vi "主界面.vi"() -> ()   [LabVIEW 2016, in "main.lvlib"]
uses:
  main.lvlib
  <vilib>/Utility/miscctls.llb/LVPointTypeDef.ctl
  <vilib>/Plasmionique/MB Master/MB_Master/MB_Master.lvclass
  DST800/DST800.lvlib
  elevator/elevator.lvlib
  EXO2/EXO2.lvlib
  DAM395CF/DAM395CF.lvlib
  <vilib>/ptbypt/NI_PtbyPt.lvlib
  bbe/bbe.lvlib
  NAQ_DO/NAQ_DO.lvlib
panel:
  out "循环次数":u32
  in  "急停按钮":bool
  out "告警信息":string
  out "运行状态":bool
  out "位置变化值":dbl
  out "编码器计数值":u16
  in  "停止按钮":bool
  in  "启动":bool
  in  "剖面视图":bool
  out "日志":string
  in  "监测数据":i32(listbox)
  out "声纳通讯":bool
  out "仪器通讯":bool
  out "IO通讯":bool
  out "多参数电源":bool caption="仪器电源"
  out "剖面下降":bool
  out "剖面上升":bool
  in  "调试":bool
  in  "设置":bool
  out "仪器位置":dbl format="%#_6f m"
  out "湖面水深":dbl format="%#_6f m"
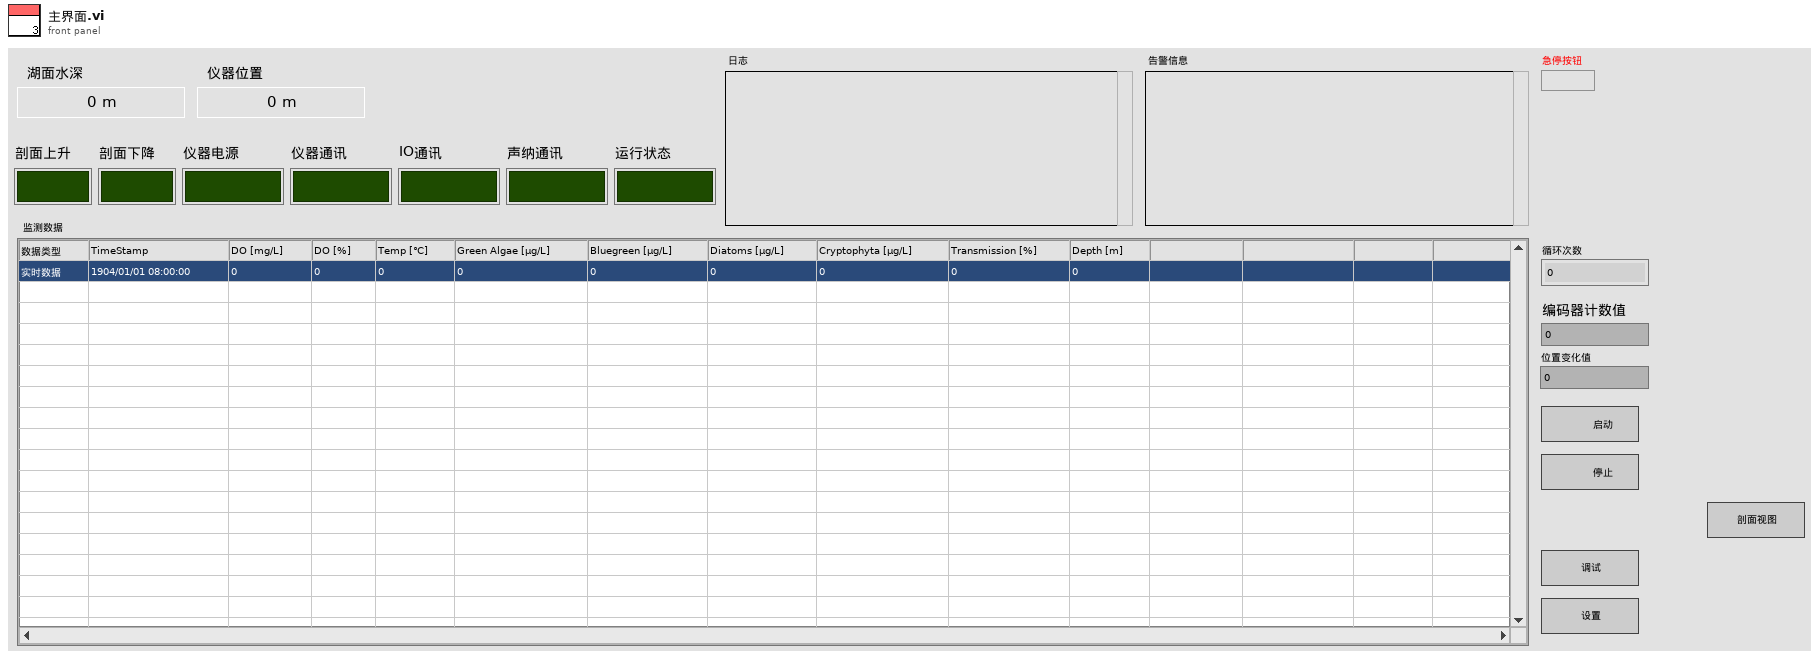
[diagram p1: front panel]
types:
  T1 = enum16{"open", "poll", "close", "run", "stop", "shutdown"}
  T2 = typedef "LVPointTypeDef.ctl" = cluster{"Horizontal":i16, "Vertical":i16}
  T3 = cluster{"Time":timestamp, "Temp":dbl, "SpCond":dbl, "Cond":dbl, "Sal":dbl, "TDS":dbl, "pH":dbl, "pH mV":dbl, "orp":dbl, "ODO %":dbl, "ODO mg/L":dbl, "Turb":dbl, "Chl":dbl, "Depth":dbl}
  T4 = cluster{"时间":timestamp, "Temp [℃]":dbl, "Green Algae [μg/L]":dbl, "Bluegreen [μg/L]":dbl, "Diatoms [μg/L]":dbl, "Cryptophyta [μg/L]":dbl, "Transmission [%]":dbl, "Depth [m]":dbl}
  T5 = cluster{"编码器工程变换系数_计数值":dbl, "编码器工程变换系数_工程值":dbl}
  T6 = typedef "checkbox.ctl" = bool
  T7 = typedef "剖面数据_EXO2.ctl" = cluster{"时间":timestamp, "测量模式":string, "数据类型":string, "数据标识":string, "湖面水深":sgl, "缆绳下放长度":sgl, "层数":u16, "row":u16, "水温":sgl, "比电导率":sgl, "电导率":sgl, "盐度":sgl, "总溶解固体":sgl, "pH":sgl, "pHmV":sgl, "ORP":sgl, "饱和度":sgl, "DO":sgl, "浊度":sgl, "叶绿素a":sgl, "水深":sgl}
  T8 = typedef "剖面数据_bbe_NAQDO.ctl" = cluster{"时间":timestamp, "测量模式":string, "数据类型":string, "数据标识":string, "湖面水深":sgl, "缆绳下放长度":sgl, "层数":u16, "row":u16, "水温":sgl, "DO":sgl, "饱和度":sgl, "绿藻":sgl, "蓝藻":sgl, "硅甲藻":sgl, "隐藻":sgl, "透光率":sgl, "水深":sgl}
  T9 = cluster{"水温":sgl, "比电导率":sgl, "电导率":sgl, "盐度":sgl, "总溶解固体":sgl, "pH":sgl, "pHmV":sgl, "ORP":sgl, "饱和度":sgl, "DO":sgl, "浊度":sgl, "叶绿素a":sgl, "水深":sgl}
  T10 = cluster{"时间标识":timestamp, "DO [mg/L]":dbl, "DO [%]":dbl}
  T11 = cluster{"水温":sgl, "DO":sgl, "饱和度":sgl, "绿藻":sgl, "蓝藻":sgl, "硅甲藻":sgl, "隐藻":sgl, "透光率":sgl, "水深":sgl}
  T12 = typedef "LVDateTimeRec.ctl" = cluster{"秒数的小数部分":dbl, "秒":i32, "分":i32, "时":i32, "日":i32, "月":i32, "年":i32, "天数（周）":i32, "天数（年）":i32, "DST":i32}
  T13 = cluster{"baud rate (bps)":u32, "stop bits":u16, "parity":u16, "flow control":u16, "timeout":u32, "retries":i32}
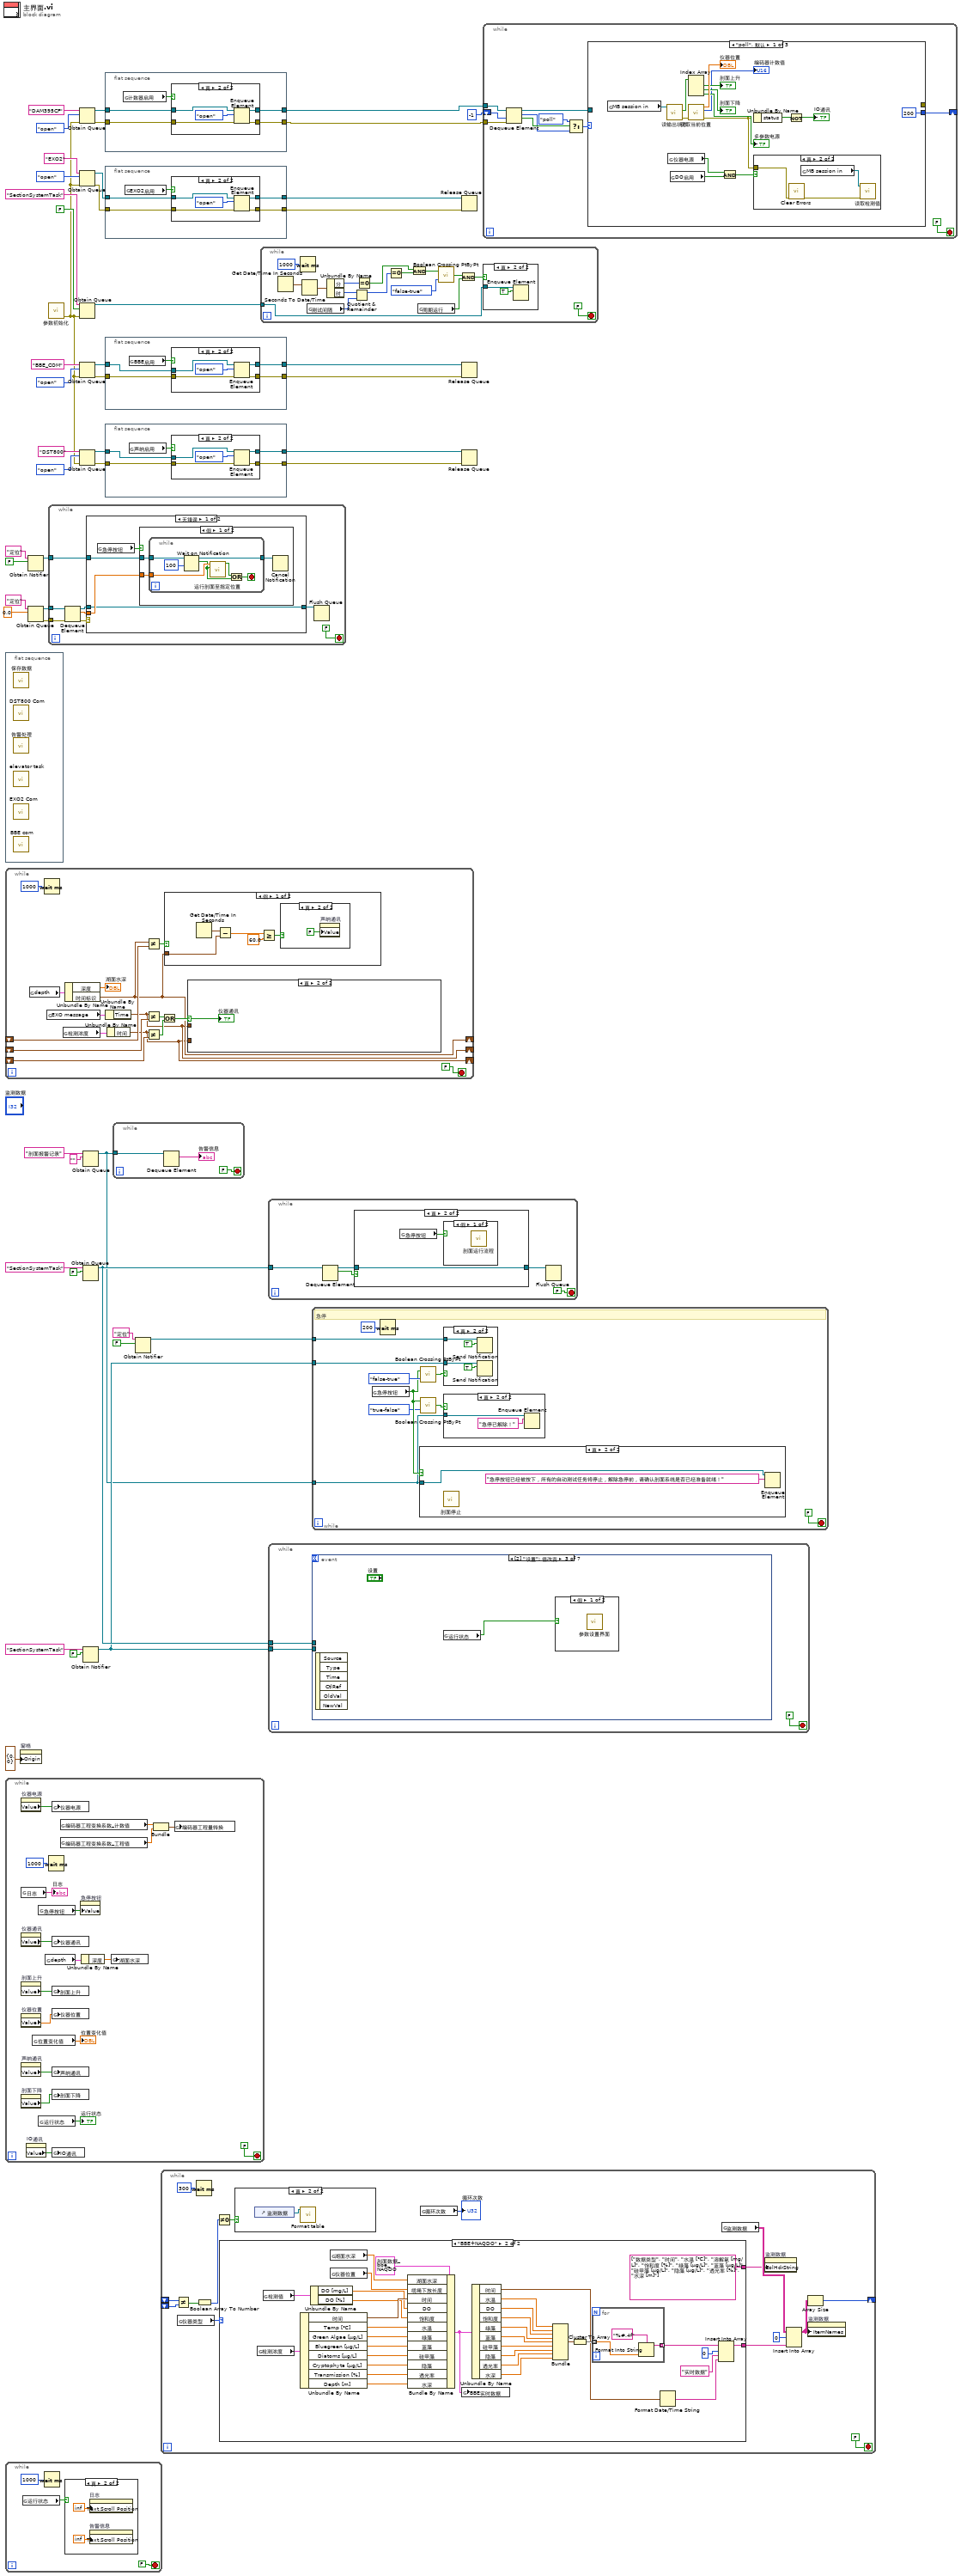
[diagram p0: block diagram]
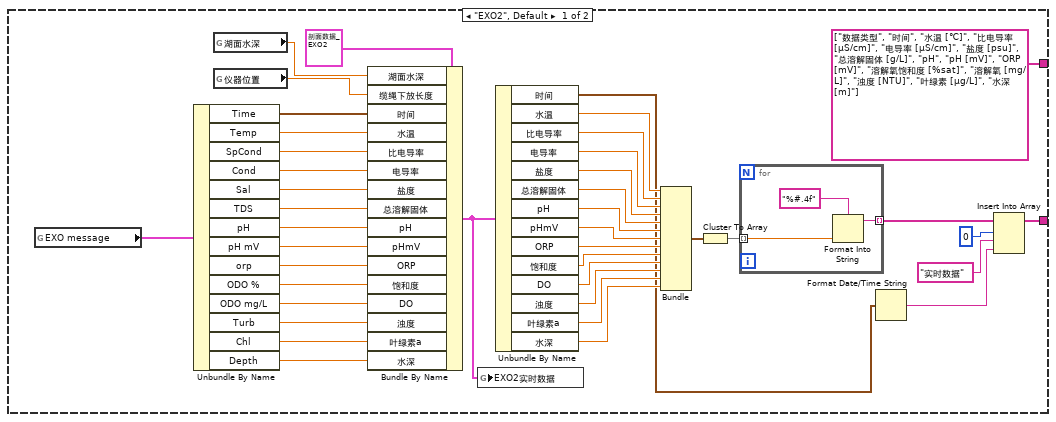
[diagram p6: hidden frame]
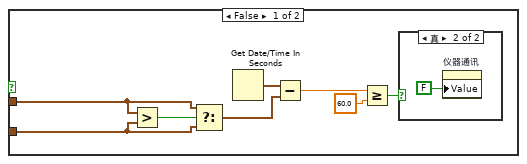
[diagram p14: hidden frame]
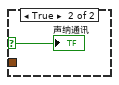
[diagram p17: hidden frame]
diagram:
  n1 = flat-sequence {
    frame #0 {
      n2 = call "保存数据.vi"() -> ()  [unwired: 12 in]
      n3 = call "DST800 Com.vi"() -> ()  [unwired: 12 in]
      n4 = call "告警处理.vi"() -> ()  [unwired: 12 in]
      n5 = call "elevator task.vi"() -> ()  [unwired: 12 in]
      n6 = call "EXO2 Com.vi"() -> ()  [unwired: 12 in]
      n7 = call "BBE com.vi"() -> ()  [unwired: 12 in]
    }
  }
  n8 = while {
    shift-right: [w52] -> _
    shift-left: _ -> [w62]
    shift-right: [w51] -> _
    shift-left: _ -> [w59]
    shift-right: [w50] -> _
    shift-left: _ -> [w56]
    stop <- FALSE stop-if-true
    n9 = global read "DST800全局变量.vi" "depth"() -> (w64:cluster{"时间标识":timestamp, "深度":dbl})
    n10 = Wait (ms)(milliseconds to wait=u32 1000 ("等待时间（毫秒）")) -> ()  [unwired: 1 out]
    n11 = global read "EXO2全局变量.vi" "EXO message"() -> (w60:T3)
    n12 = global read "过程变量.vi" "检测浓度"() -> (w57:T4)
    n13 = Unbundle By Name(w64) -> ("深度"=→"湖面水深":dbl, "时间标识"=w52:timestamp)
    n14 = Unbundle By Name(w60) -> ("Time"=w51:timestamp)
    n15 = Unbundle By Name(w57) -> ("时间"=w50:timestamp)
    n16 = Not Equal?(x=w52, y=w62) -> (x != y?=w54:bool)
    n17 = Not Equal?(x=w51, y=w59) -> (x != y?=w58:bool)
    n18 = Not Equal?(x=w50, y=w56) -> (x != y?=w55:bool)
    n19 = Or(x=w58, y=w55) -> (x .or. y?=w53:bool)
    n20 = case shown="假" w54 {
      selector: w54 -> [_ w82]
      tunnel: w52 -> [w80 _]
      frame False {
        n21 = Get Date/Time In Seconds() -> (seconds since 1Jan1904=w79:timestamp)
        n22 = Subtract(x=w79, y=w80) -> (x-y=w78:dbl)
        n23 = Greater Or Equal?(x=w78, y=60.0) -> (x >= y?=w76:bool)
        n24 = case shown="真" w76 {
          frame False {
          }
          frame True {
            n25 = property on="声纳通讯" class="Bool (严格)"("Value"=FALSE ("声纳通讯")) -> ()  [unwired: 2 in, 2 out]
          }
        }
      }
      frame True {
        "声纳通讯" <- w82
      }
    }
    n26 = case shown="真" w53 {
      selector: w53 -> [_ w75]
      tunnel: w51 -> [w68 _]
      tunnel: w50 -> [w67 _]
      frame False {
        n27 = Greater?(x=w68, y=w67) -> (0:w69:bool)
        n28 = Select(t=w68, s=w69, f=w67) -> (s? t:f=w66:timestamp)
        n29 = Get Date/Time In Seconds() -> (seconds since 1Jan1904=w70:timestamp)
        n30 = Subtract(x=w70, y=w66) -> (x-y=w71:dbl)
        n31 = Greater Or Equal?(x=w71, y=60.0) -> (x >= y?=w73:bool)
        n32 = case shown="真" w73 {
          frame False {
          }
          frame True {
            n33 = property on="仪器通讯" class="Bool (严格)"("Value"=FALSE ("声纳通讯")) -> ()  [unwired: 2 in, 2 out]
          }
        }
      }
      frame True {
        "仪器通讯" <- w75
      }
    }
  }
  n34 = while {
    stop <- FALSE stop-if-true
    n35 = property on="仪器电源" class="Bool (严格)"() -> ("Value"=w84:bool)  [unwired: 2 in, 2 out]
    n36 = global read "全局非断电保持变量.vi" "日志"() -> (→"日志":string)
    n37 = property on="仪器通讯" class="Bool (严格)"() -> ("Value"=w93:bool)  [unwired: 2 in, 2 out]
    n38 = property on="剖面上升" class="Bool (严格)"() -> ("Value"=w95:bool)  [unwired: 2 in, 2 out]
    n39 = property on="仪器位置" class="DigNum (严格)"() -> ("Value"=w92:dbl)  [unwired: 2 in, 2 out]
    n40 = property on="声纳通讯" class="Bool (严格)"() -> ("Value"=w94:bool)  [unwired: 2 in, 2 out]
    n41 = property on="剖面下降" class="Bool (严格)"() -> ("Value"=w96:bool)  [unwired: 2 in, 2 out]
    n42 = property on="IO通讯" class="Bool (严格)"() -> ("Value"=w97:bool)  [unwired: 2 in, 2 out]
    n43 = global read "全局非断电保持变量.vi" "位置变化值"() -> (→"位置变化值":dbl)
    n44 = global read "全局非断电保持变量.vi" "急停按钮"() -> (w83:bool)
    n45 = global read "全局非断电保持变量.vi" "运行状态"() -> (→"运行状态":bool)
    n46 = global read "DST800全局变量.vi" "depth"() -> (w99:cluster{"时间标识":timestamp, "深度":dbl})
    n47 = Wait (ms)(milliseconds to wait=u32 1000 ("等待时间（毫秒）")) -> ()  [unwired: 1 out]
    n48 = global write "全局非断电保持变量.vi" "仪器电源"(w84) -> ()
    n49 = global write "全局非断电保持变量.vi" "仪器通讯"(w93) -> ()
    n50 = global write "全局非断电保持变量.vi" "剖面上升"(w95) -> ()
    n51 = global write "全局非断电保持变量.vi" "仪器位置"(w92) -> ()
    n52 = global write "全局非断电保持变量.vi" "声纳通讯"(w94) -> ()
    n53 = global write "全局非断电保持变量.vi" "剖面下降"(w96) -> ()
    n54 = global write "全局非断电保持变量.vi" "IO通讯"(w97) -> ()
    n55 = global read "全局断电保存变量.vi" "编码器工程变换系数_计数值"() -> (w89:dbl)
    n56 = global read "全局断电保存变量.vi" "编码器工程变换系数_工程值"() -> (w88:dbl)
    n57 = property on="急停按钮" class="Bool (严格)"("Value"=w83) -> ()  [unwired: 2 in, 2 out]
    n58 = Unbundle By Name(w99) -> ("深度"=w98:dbl)
    n59 = global write "全局非断电保持变量.vi" "湖面水深"(w98) -> ()
    n60 = Bundle("编码器工程变换系数_计数值"=w89, "编码器工程变换系数_工程值"=w88) -> (w87:T5)  [unwired: 1 in]
    n61 = global write "elevator 全局变量.vi" "编码器工程量转换"(w87) -> ()
  }
  n62 = while {
    stop <- FALSE stop-if-true
    n63 = global read "全局非断电保持变量.vi" "运行状态"() -> (w101:bool)
    n64 = Wait (ms)(milliseconds to wait=u32 1000 ("等待时间（毫秒）")) -> ()  [unwired: 1 out]
    n65 = case shown="真" w101 {
      frame False {
      }
      frame True {
        n66 = property on="日志" class="Str"("Text.Scroll Position"=inf) -> ()  [unwired: 2 in, 2 out]
        n67 = property on="告警信息" class="Str"("Text.Scroll Position"=inf) -> ()  [unwired: 2 in, 2 out]
      }
    }
  }
  n68 = property on="窗格" class="Pane"("Origin"=T2 {"Horizontal"=0, "Vertical"=0} ("原点")) -> ()  [unwired: 2 in, 2 out]
  n69 = Obtain Notifier(name (unnamed)="定位" ("名称（未命名）"), notification data type=FALSE) -> (notifier out=w18:refnum<notifier>)  [unwired: 2 in, 2 out]
  n70 = Obtain Queue(name (unnamed)="定位" ("名称（未命名）"), element data type=0.0) -> (queue out=w22:refnum<queue>, error out=w21:errorcluster)  [unwired: 3 in, 1 out]
  n71 = call "参数初始化.vi"() -> ("error out"=w6:errorcluster)  [unwired: 11 in]
  n72 = while {
    tunnel: w22 -> [w113]
    tunnel: w21 -> [w112]
    tunnel: w18 -> [w109]
    stop <- FALSE stop-if-true
    n73 = Dequeue Element(queue=w113, error in (no error)=w112) -> (queue out=w108:refnum<queue>, element=w110:dbl, error out=w111:errorcluster)  [unwired: 1 in, 1 out]
    n74 = case shown="无错误" w111 {
      tunnel: w110 -> [w117 _]
      tunnel: w109 -> [w116 _]
      tunnel: [w115 w128] -> w107
      tunnel: w108 -> [w115 w128]
      frame No Error {
        n75 = global read "全局非断电保持变量.vi" "急停按钮"() -> (w114:bool)
        n76 = case shown="假" w114 {
          tunnel: w117 -> [w120 _]
          tunnel: w116 -> [w119 _]
          frame False {
            n77 = while {
              tunnel: w120 -> [w127]
              tunnel: w119 -> [w126]
              tunnel: [w122] -> w118
              stop <- w124 stop-if-true
              n78 = Wait on Notification(notifier=w126, timeout in ms (-1)=100 ("超时毫秒(-1)")) -> (notifier out=w122:refnum<notifier>, notification=w121:bool)  [unwired: 2 in, 2 out]
              n79 = call "运行剖面至指定位置.vi"("停止"=w121, "位置设置值"=w127) -> ("定位完成"=w123:bool)  [unwired: 8 in, 1 out]
              n80 = Or(x=w123, y=w121) -> (x .or. y?=w124:bool)
            }
            n81 = Cancel Notification(0:w118) -> ()  [unwired: 1 in, 3 out]
          }
          frame True {
          }
        }
      }
      frame Error {
      }
    }
    n82 = Flush Queue(queue=w107) -> ()  [unwired: 1 in, 3 out]
  }
  n83 = Obtain Queue(name (unnamed)="DAM395CF" ("名称（未命名）"), element data type=enum16{"open", "close", "poll"}."open" ("枚举"), error in (no error)=w6) -> (queue out=w34:refnum<queue>, error out=w32:errorcluster)  [unwired: 2 in, 1 out]
  n84 = Obtain Queue(name (unnamed)="EXO2" ("名称（未命名）"), element data type=T1."open" ("枚举"), error in (no error)=w6) -> (queue out=w37:refnum<queue>, error out=w40:errorcluster)  [unwired: 2 in, 1 out]
  n85 = Obtain Queue(name (unnamed)="SectionSystemTask" ("名称（未命名）"), element data type=FALSE, error in (no error)=w6) -> (queue out=w13:refnum<queue>)  [unwired: 2 in, 2 out]
  n86 = Obtain Queue(name (unnamed)="BBE_COM" ("名称（未命名）"), element data type=enum16{"open", "close", "poll"}."open" ("枚举"), error in (no error)=w6) -> (queue out=w8:refnum<queue>, error out=w7:errorcluster)  [unwired: 2 in, 1 out]
  n87 = Obtain Queue(name (unnamed)="DST800" ("名称（未命名）"), element data type=enum16{"open", "poll", "close", "shutdown"}."open" ("枚举"), error in (no error)=w6) -> (queue out=w44:refnum<queue>, error out=w41:errorcluster)  [unwired: 2 in, 1 out]
  n88 = Obtain Queue(name (unnamed)="SectionSystemTask" ("名称（未命名）"), element data type=FALSE) -> (queue out=w28:refnum<queue>)  [unwired: 3 in, 2 out]
  n89 = Obtain Notifier(name (unnamed)="SectionSystemTask" ("名称（未命名）"), notification data type=FALSE) -> (notifier out=w5:refnum<notifier>)  [unwired: 2 in, 2 out]
  n90 = Obtain Queue(name (unnamed)="剖面报警记录" ("名称（未命名）"), element data type="") -> (queue out=w4:refnum<queue>)  [unwired: 3 in, 2 out]
  n91 = flat-sequence {
    tunnel: w34 -> [w133]
    tunnel: [w131] -> w33
    tunnel: [w130] -> w31
    tunnel: w32 -> [w129]
    frame #0 {
      n92 = global read "全局断电保存变量.vi" "计数器启用"() -> (w132:T6)
      n93 = case shown="真" w132 {
        tunnel: w133 -> [w135 w140]
        tunnel: [w135 w139] -> w131
        tunnel: [w134 w138] -> w130
        tunnel: w129 -> [w134 w137]
        frame False {
        }
        frame True {
          n94 = Enqueue Element(queue=w140, element=enum16{"open", "close", "poll"}."open" ("枚举"), error in (no error)=w137) -> (queue out=w139:refnum<queue>, error out=w138:errorcluster)  [unwired: 1 in, 1 out]
        }
      }
    }
  }
  n95 = flat-sequence {
    tunnel: w37 -> [w145]
    tunnel: [w143] -> w38
    tunnel: [w142] -> w39
    tunnel: w40 -> [w141]
    frame #0 {
      n96 = global read "全局断电保存变量.vi" "EXO2启用"() -> (w144:T6)
      n97 = case shown="真" w144 {
        tunnel: w145 -> [w147 w152]
        tunnel: [w147 w151] -> w143
        tunnel: [w146 w150] -> w142
        tunnel: w141 -> [w146 w149]
        frame False {
        }
        frame True {
          n98 = Enqueue Element(queue=w152, element=T1."open" ("枚举"), error in (no error)=w149) -> (queue out=w151:refnum<queue>, error out=w150:errorcluster)  [unwired: 1 in, 1 out]
        }
      }
    }
  }
  n99 = flat-sequence {
    tunnel: [w156] -> w9
    tunnel: [w155] -> w10
    tunnel: w7 -> [w154]
    tunnel: w8 -> [w153]
    frame #0 {
      n100 = global read "全局断电保存变量.vi" "BBE启用"() -> (w157:T6)
      n101 = case shown="真" w157 {
        tunnel: w153 -> [w159 w164]
        tunnel: [w159 w163] -> w156
        tunnel: [w158 w162] -> w155
        tunnel: w154 -> [w158 w161]
        frame False {
        }
        frame True {
          n102 = Enqueue Element(queue=w164, element=enum16{"open", "close", "poll"}."open" ("枚举"), error in (no error)=w161) -> (queue out=w163:refnum<queue>, error out=w162:errorcluster)  [unwired: 1 in, 1 out]
        }
      }
    }
  }
  n103 = flat-sequence {
    tunnel: w44 -> [w169]
    tunnel: [w167] -> w43
    tunnel: [w166] -> w42
    tunnel: w41 -> [w165]
    frame #0 {
      n104 = global read "全局断电保存变量.vi" "声纳启用"() -> (w168:T6)
      n105 = case shown="真" w168 {
        tunnel: w169 -> [w171 w176]
        tunnel: [w171 w174] -> w167
        tunnel: [w170 w173] -> w166
        tunnel: w165 -> [w170 w172]
        frame False {
        }
        frame True {
          n106 = Enqueue Element(queue=w176, element=enum16{"open", "poll", "close", "shutdown"}."open" ("元素"), error in (no error)=w172) -> (queue out=w174:refnum<queue>, error out=w173:errorcluster)  [unwired: 1 in, 1 out]
        }
      }
    }
  }
  n107 = while {
    tunnel: w4 -> [w179]
    stop <- FALSE stop-if-true
    n108 = Dequeue Element(queue=w179) -> (element=→"告警信息":string)  [unwired: 2 in, 3 out]
  }
  n109 = Obtain Notifier(name (unnamed)="定位" ("名称（未命名）"), notification data type=FALSE) -> (notifier out=w1:refnum<notifier>)  [unwired: 2 in, 2 out]
  n110 = while {
    shift-right: [w182] -> _
    shift-left: _ -> [w187]
    shift-left: _ -> [w186]
    stop <- FALSE stop-if-true
    n111 = Not Equal?(x=w187, y=w186) -> (x != y?=w181:bool[])
    n112 = global read "全局断电保存变量.vi" "仪器类型"() -> (w190:enum16{"EXO2", "BBE+NAQDO"})
    n113 = Wait (ms)(milliseconds to wait=u32 300 ("等待时间（毫秒）")) -> ()  [unwired: 1 out]
    n114 = Boolean Array To Number(Boolean array=w181) -> (number=w185:u32)
    n115 = Not Equal To 0?(x=w185) -> (x != 0?=w184:bool)
    n116 = case shown="\"BBE+NAQDO\"" w190 {
      tunnel: [string[] ["数据类型", "时间", "水温 [℃]", "比电导率 [μS/cm]", "电导率 [μS/cm]", "盐度 [psu]", "总溶解固体 [g/L]", "pH", "pH [mV]", "ORP [mV]", "溶解氧饱和度 [%sat]", "溶解氧 [mg/L]", "浊度 [NTU]", "叶绿素 [μg/L]", "水深 [m]"] ("列首字符串[]") string[] ["数据类型", "时间", "水温 [℃]", "溶解氧 [mg/L]", "饱和度 [%]", "绿藻 [μg/L]", "蓝藻 [μg/L]", "硅甲藻 [μg/L]", "隐藻 [μg/L]", "透光率 [%]", "水深 [m]"] ("列首字符串[]")] -> w188
      tunnel: [w230 w267] -> w189
      frame "EXO2", Default {
        n117 = global read "EXO2全局变量.vi" "EXO message"() -> (w213:T3)
        n118 = Unbundle By Name(w213) -> ("Time"=w227:timestamp, "Temp"=w214:dbl, "SpCond"=w215:dbl, "Cond"=w216:dbl, "Sal"=w217:dbl, "TDS"=w218:dbl, "pH"=w219:dbl, "pH mV"=w220:dbl, "orp"=w221:dbl, "ODO %"=w222:dbl, "ODO mg/L"=w223:dbl, "Turb"=w224:dbl, "Chl"=w225:dbl, "Depth"=w226:dbl)
        n119 = global read "全局非断电保持变量.vi" "湖面水深"() -> (w228:dbl)
        n120 = global read "全局非断电保持变量.vi" "仪器位置"() -> (w229:dbl)
        n121 = Bundle By Name(cluster=T7 {"时间"=timestamp(0 s since 1904-01-01), "测量模式"="水样测试", "数据类型"="N", "数据标识"="N", "湖面水深"=0.0, "缆绳下放长度"=0.0, "层数"=0, "row"=0, "水温"=0.0, "比电导率"=0.0, "电导率"=0.0, "盐度"=0.0, "总溶解固体"=0.0, "pH"=0.0, "pHmV"=0.0, "ORP"=0.0, "饱和度"=0.0, "DO"=0.0, "浊度"=0.0, "叶绿素a"=0.0, "水深"=0.0} ("data"), "湖面水深"=w228, "缆绳下放长度"=w229, "时间"=w227, "水温"=w214, "比电导率"=w215, "电导率"=w216, "盐度"=w217, "总溶解固体"=w218, "pH"=w219, "pHmV"=w220, "ORP"=w221, "饱和度"=w222, "DO"=w223, "浊度"=w224, "叶绿素a"=w225, "水深"=w226) -> (w196:T7)
        n122 = global write "全局非断电保持变量.vi" "EXO2实时数据"(w196) -> ()
        n123 = Unbundle By Name(w196) -> ("时间"=w198:timestamp, "水温"=w211:sgl, "比电导率"=w210:sgl, "电导率"=w209:sgl, "盐度"=w208:sgl, "总溶解固体"=w207:sgl, "pH"=w206:sgl, "pHmV"=w205:sgl, "ORP"=w204:sgl, "饱和度"=w203:sgl, "DO"=w202:sgl, "浊度"=w201:sgl, "叶绿素a"=w200:sgl, "水深"=w199:sgl)
        n124 = Bundle("水温"=w211, "比电导率"=w210, "电导率"=w209, "盐度"=w208, "总溶解固体"=w207, "pH"=w206, "pHmV"=w205, "ORP"=w204, "饱和度"=w203, "DO"=w202, "浊度"=w201, "叶绿素a"=w200, "水深"=w199) -> (w197:T9)  [unwired: 1 in]
        n125 = Cluster To Array(cluster=w197) -> (array=w235:sgl[])
        n126 = for {
          tunnel: w235 -> [w239] mode=indexing
          tunnel: [w237] -> w234 mode=indexing
          n127 = Format Into String(format string="%#.4f" ("格式字符串"), w239) -> (resulting string=w237:string)  [unwired: 2 in, 1 out]
        }
        n128 = Format Date/Time String(seconds (now)=w198) -> (date/time string=w233:string)  [unwired: 2 in]
        n129 = Insert Into Array(array=w234, index=0 ("索引"), new element #1="实时数据" ("格式字符串"), new element #2=w233) -> (w230:string[])
      }
      frame "BBE+NAQDO" {
        n130 = global read "过程变量.vi" "检测浓度"() -> (w252:T4)
        n131 = global read "过程变量.vi" "检测值"() -> (w253:T10)
        n132 = Unbundle By Name(w252) -> ("时间"=w256:timestamp, "Temp [℃]"=w257:dbl, "Green Algae [μg/L]"=w258:dbl, "Bluegreen [μg/L]"=w259:dbl, "Diatoms [μg/L]"=w260:dbl, "Cryptophyta [μg/L]"=w261:dbl, "Transmission [%]"=w262:dbl, "Depth [m]"=w263:dbl)
        n133 = Unbundle By Name(w253) -> ("DO [mg/L]"=w254:dbl, "DO [%]"=w255:dbl)
        n134 = global read "全局非断电保持变量.vi" "湖面水深"() -> (w266:dbl)
        n135 = global read "全局非断电保持变量.vi" "仪器位置"() -> (w265:dbl)
        n136 = Bundle By Name(cluster=T8 {"时间"=timestamp(0 s since 1904-01-01), "测量模式"="水样测试", "数据类型"="N", "数据标识"="N", "湖面水深"=0.0, "缆绳下放长度"=0.0, "层数"=0, "row"=0, "水温"=0.0, "DO"=0.0, "饱和度"=0.0, "绿藻"=0.0, "蓝藻"=0.0, "硅甲藻"=0.0, "隐藻"=0.0, "透光率"=0.0, "水深"=0.0} ("columns"), "湖面水深"=w266, "缆绳下放长度"=w265, "时间"=w256, "DO"=w254, "饱和度"=w255, "水温"=w257, "绿藻"=w258, "蓝藻"=w259, "硅甲藻"=w260, "隐藻"=w261, "透光率"=w262, "水深"=w263) -> (w240:T8)
        n137 = global write "全局非断电保持变量.vi" "BBE实时数据"(w240) -> ()
        n138 = Unbundle By Name(w240) -> ("时间"=w251:timestamp, "水温"=w250:sgl, "DO"=w249:sgl, "饱和度"=w248:sgl, "绿藻"=w247:sgl, "蓝藻"=w246:sgl, "硅甲藻"=w245:sgl, "隐藻"=w244:sgl, "透光率"=w243:sgl, "水深"=w242:sgl)
        n139 = Bundle("水温"=w250, "DO"=w249, "饱和度"=w248, "绿藻"=w247, "蓝藻"=w246, "硅甲藻"=w245, "隐藻"=w244, "透光率"=w243, "水深"=w242) -> (w241:T11)  [unwired: 1 in]
        n140 = Cluster To Array(cluster=w241) -> (array=w268:sgl[])
        n141 = for {
          tunnel: w268 -> [w276] mode=indexing
          tunnel: [w274] -> w272 mode=indexing
          n142 = Format Into String(format string="%#.4f" ("格式字符串"), w276) -> (resulting string=w274:string)  [unwired: 2 in, 1 out]
        }
        n143 = Format Date/Time String(seconds (now)=w251) -> (date/time string=w271:string)  [unwired: 2 in]
        n144 = Insert Into Array(array=w272, index=0 ("索引"), new element #1="实时数据" ("格式字符串"), new element #2=w271) -> (w267:string[])
      }
    }
    n145 = case shown="真" w184 {
      frame False {
      }
      frame True {
        n146 = control-ref of="监测数据"() -> (w195:refnum<vi>)
        n147 = call "Format table.vi"("Table输入"=w195) -> ()  [unwired: 11 in]
      }
    }
    n148 = global read "全局非断电保持变量.vi" "循环次数"() -> (→"循环次数":u32)
    n149 = global read "全局非断电保持变量.vi" "监测数据"() -> (w191:string[][])
    n150 = property on="监测数据" class="MCListbox (严格)"("ColHdrString"=w188) -> ()  [unwired: 2 in, 2 out]
    n151 = Insert Into Array(array=w191, index (row)=0 ("索引 (行)"), new element=w189) -> (w183:string[][])  [unwired: 1 in]
    n152 = Array Size(array=w183) -> (size(s)=w182:i32[])
    n153 = property on="监测数据" class="MCListbox (严格)"("ItemNames"=w183) -> ()  [unwired: 2 in, 2 out]
  }
  n154 = while {
    tunnel: w13 -> [w284]
    stop <- FALSE stop-if-true
    n155 = Get Date/Time In Seconds() -> (seconds since 1Jan1904=w291:timestamp)
    n156 = Wait (ms)(milliseconds to wait=u32 1000 ("等待时间（毫秒）")) -> ()  [unwired: 1 out]
    n157 = Seconds To Date/Time(time stamp (now)=w291) -> (date time rec=w290:T12)  [unwired: 1 in]
    n158 = global read "全局断电保存变量.vi" "测试间隔"() -> (w278:u16)
    n159 = Unbundle By Name(w290) -> ("分"=w287:i32, "时"=w289:i32)
    n160 = Quotient & Remainder(x=w289, y=w278) -> (x-y*floor(x/y)=w288:i32)  [unwired: 1 out]
    n161 = Equal To 0?(x=w287) -> (x = 0?=w285:bool)
    n162 = Equal To 0?(x=w288) -> (x = 0?=w286:bool)
    n163 = And(x=w285, y=w286) -> (x .and. y?=w283:bool)
    n164 = global read "全局断电保存变量.vi" "周期运行"() -> (w277:bool)
    n165 = call <vilib>:"Boolean Crossing PtByPt.vi"("direction"=enum16{"either", "false-true", "true-false"}."false-true", "input"=w283) -> ("crossing"=w281:bool)  [unwired: 1 in]
    n166 = And(x=w281, y=w277) -> (x .and. y?=w282:bool)
    n167 = case shown="真" w282 {
      tunnel: w284 -> [_ w294]
      frame False {
      }
      frame True {
        n168 = Enqueue Element(queue=w294, element=TRUE ("元素")) -> ()  [unwired: 2 in, 3 out]
      }
    }
  }
  n169 = while {
    tunnel: w28 -> [w299]
    stop <- FALSE stop-if-true
    n170 = Dequeue Element(queue=w299) -> (queue out=w297:refnum<queue>, element=w298:bool)  [unwired: 2 in, 2 out]
    n171 = case shown="真" w298 {
      tunnel: [w300 w302] -> w296
      tunnel: w297 -> [w300 w302]
      frame False {
      }
      frame True {
        n172 = global read "全局非断电保持变量.vi" "急停按钮"() -> (w301:bool)
        n173 = case shown="假" w301 {
          frame False {
            n174 = call "剖面运行流程.vi"() -> ()  [unwired: 12 in]
          }
          frame True {
          }
        }
      }
    }
    n175 = Flush Queue(queue=w296) -> ()  [unwired: 1 in, 3 out]
  }
  n176 = while {
    tunnel: w28 -> [w304]
    tunnel: w5 -> [w303]
    stop <- FALSE stop-if-true
    n177 = event shown="[2] \"设置\": 值改变" {
      selector: _ -> [_ _ _ _ _ _ _]
      dyn-events: _ -> [_ _ _ _ _ _ _]
      timeout: _ -> [_ _ _ _ _ _ _]
      tunnel: w304 -> [_ _ _ _ w319 _ _]
      tunnel: w303 -> [_ _ _ _ _ w321 _]
      event Timeout {
        n178 = event-data() -> ()  [unwired: 1 in, 3 out]
      }
      event "急停按钮": Value Change {
        n179 = event-data() -> ("OldVal"=w308:bool)  [unwired: 1 in, 5 out]
        n180 = case shown="真" w308 {
          tunnel: [TRUE ("T button?") w313] -> w307
          tunnel: [TRUE w312] -> w306
          frame False {
          }
          frame True {
            n181 = Two Button Dialog(message="解除急停前，请确认剖面系统是否已经准备就绪！" ("消息")) -> (T button?=w313:bool)  [unwired: 2 in]
            n182 = Not(x=w313) -> (.not. x?=w312:bool)
          }
        }
        n183 = case shown="真" w307 {
          tunnel: w306 -> [_ w309]
          frame False {
          }
          frame True {
            n184 = global write "全局非断电保持变量.vi" "急停按钮"(w309) -> ()
          }
        }
      }
      event "设置": Value Change {
        n185 = event-data() -> ()  [unwired: 1 in, 6 out]
        n186 = global read "全局非断电保持变量.vi" "运行状态"() -> (w315:bool)
        n187 = case shown="假" w315 {
          frame False {
            n188 = call "参数设置界面.vi"() -> ()  [unwired: 12 in]
          }
          frame True {
          }
        }
      }
      event "调试": Value Change {
        n189 = event-data() -> ()  [unwired: 1 in, 6 out]
        n190 = global read "全局非断电保持变量.vi" "运行状态"() -> (w316:bool)
        n191 = case shown="假" w316 {
          frame False {
            n192 = call "调试画面.vi"() -> ()  [unwired: 12 in]
          }
          frame True {
          }
        }
      }
      event "启动": Value Change {
        n193 = event-data() -> ()  [unwired: 1 in, 1 out]
        n194 = Two Button Dialog(message="请确认剖面仪器是否已投入水中，否则剖面系统将工作异常！" ("消息")) -> (T button?=w317:bool)  [unwired: 2 in]
        n195 = Enqueue Element(queue=w319, element=w317) -> ()  [unwired: 2 in, 3 out]
      }
      event "停止按钮": Value Change {
        n196 = event-data() -> ()  [unwired: 1 in, 1 out]
        n197 = Send Notification(notification=TRUE ("通知"), notifier=w321) -> ()  [unwired: 1 in, 2 out]
      }
      event "剖面视图": Value Change {
        n198 = event-data() -> ()  [unwired: 1 in, 6 out]
        n199 = call "剖面视图.vi"() -> ()  [unwired: 12 in]
      }
    }
  }
  n200 = while {
    tunnel: w5 -> [w328]
    tunnel: w4 -> [w323]
    tunnel: w1 -> [w322]
    stop <- FALSE stop-if-true
    # "急停"
    n201 = global read "全局非断电保持变量.vi" "急停按钮"() -> (w326:bool)
    n202 = Wait (ms)(milliseconds to wait=u32 200 ("等待时间（毫秒）")) -> ()  [unwired: 1 out]
    n203 = case shown="真" w326 {
      tunnel: w323 -> [_ w335]
      frame False {
      }
      frame True {
        n204 = call "剖面停止.vi"() -> ()  [unwired: 11 in, 1 out]
        n205 = Enqueue Element(queue=w335, element="急停按钮已经被按下，所有的自动测试任务将停止，解除急停前，请确认剖面系统是否已经准备就绪！" ("元素")) -> ()  [unwired: 2 in, 3 out]
      }
    }
    n206 = call <vilib>:"Boolean Crossing PtByPt.vi"("direction"=enum16{"either", "false-true", "true-false"}."false-true", "input"=w326) -> ("crossing"=w329:bool)  [unwired: 1 in]
    n207 = call <vilib>:"Boolean Crossing PtByPt.vi"("direction"=enum16{"either", "false-true", "true-false"}."true-false", "input"=w326) -> ("crossing"=w324:bool)  [unwired: 1 in]
    n208 = case shown="真" w329 {
      tunnel: w328 -> [_ w339]
      tunnel: w322 -> [_ w337]
      frame False {
      }
      frame True {
        n209 = Send Notification(notification=TRUE ("通知"), notifier=w337) -> ()  [unwired: 1 in, 2 out]
        n210 = Send Notification(notification=TRUE ("通知"), notifier=w339) -> ()  [unwired: 1 in, 2 out]
      }
    }
    n211 = case shown="真" w324 {
      tunnel: w323 -> [_ w333]
      frame False {
      }
      frame True {
        n212 = Enqueue Element(queue=w333, element="急停已解除！" ("元素")) -> ()  [unwired: 2 in, 3 out]
      }
    }
  }
  n213 = Release Queue(queue=w38, error in (no error)=w39) -> ()  [unwired: 1 in, 3 out]
  n214 = Release Queue(queue=w9, error in (no error)=w10) -> ()  [unwired: 1 in, 3 out]
  n215 = Release Queue(queue=w43, error in (no error)=w42) -> ()  [unwired: 1 in, 3 out]
  n216 = while {
    tunnel: w33 -> [w349]
    tunnel: w31 -> [w347]
    shift-right: [w345] -> _
    shift-left: -1 -> [w344]
    stop <- FALSE stop-if-true
    n217 = Dequeue Element(queue=w349, timeout in ms (-1)=w344, error in (no error)=w347) -> (queue out=w346:refnum<queue>, element=w342:enum16{"open", "close", "poll"}, timed out?=w343:bool)  [unwired: 1 out]
    n218 = Select(t=enum16{"open", "close", "poll"}."poll", s=w343, f=w342) -> (s? t:f=w341:enum16{"open", "close", "poll"})
    n219 = case shown="\"poll\", 默认" w341 {
      tunnel: [_ _ w380] -> _
      tunnel: w346 -> [_ _ _]
      tunnel: [200 w369 -1] -> w345
      frame "poll", Default {
        n220 = global read "elevator 全局变量.vi" "MB session in"() -> (w363:refnum<class "MB_Master.lvclass">)
        n221 = call "读输出状态.vi"("MB session in"=w363) -> ("error out"=w362:errorcluster, "Coils"=w360:bool[])  [unwired: 8 in, 1 out]
        n222 = global read "全局非断电保持变量.vi" "仪器电源"() -> (w351:bool)
        n223 = global read "全局断电保存变量.vi" "DO启用"() -> (w352:T6)
        n224 = Index Array(array=w360) -> (element #1=→"剖面上升":bool, element #2=→"剖面下降":bool, element #3=→"多参数电源":bool)  [unwired: 3 in]
        n225 = call "获取当前位置.vi"("error in (no error)"=w362) -> ("error out"=w353:errorcluster, "编码器计数值"=→"编码器计数值":u16, "编码器工程量"=→"仪器位置":dbl)  [unwired: 8 in]
        n226 = And(x=w351, y=w352) -> (x .and. y?=w350:T6)
        n227 = Unbundle By Name(w353) -> ("status"=w357:bool)
        n228 = case shown="真" w350 {
          tunnel: w353 -> [_ w367]
          frame False {
          }
          frame True {
            n229 = call <vilib>:"Clear Errors.vi"("error in (no error)"=w367) -> ("error out"=w366:errorcluster)  [unwired: 5 in, 1 out]
            n230 = global read "elevator 全局变量.vi" "MB session in"() -> (w365:refnum<class "MB_Master.lvclass">)
            n231 = call "读取检测值.vi"("error in (no error)"=w366, "MB session in"=w365) -> ()  [unwired: 9 in, 1 out]
          }
        }
        n232 = Not(x=w357) -> (.not. x?=→"IO通讯":bool)
      }
      frame "open" {
        n233 = global read "elevator 全局变量.vi" "MB session in"() -> (w372:refnum<class "MB_Master.lvclass">)
        n234 = call-dynamic "Close Session.vi"("MB session in"=w372) -> ("error out"=w371:errorcluster)  [unwired: 10 in]
        n235 = global read "全局断电保存变量.vi" "计数器串口"() -> (w376:refnum<visa-resource-name>)
        n236 = call <vilib>:"Clear Errors.vi"("error in (no error)"=w371) -> ("error out"=w370:errorcluster)  [unwired: 5 in, 1 out]
        n237 = call "open MB.vi"("Error in"=w370, "Serial Config"=T13 {"baud rate (bps)"=9600, "stop bits"=10, "parity"=0, "flow control"=0, "timeout"=1000, "retries"=1}, "Slave ID"=u8 1, "VISA Resource"=w376) -> ("Error out"=w368:errorcluster, "MB session out"=w373:refnum<class "MB_Master.lvclass">)  [unwired: 6 in]
        n238 = global write "elevator 全局变量.vi" "MB session in"(w373) -> ()
        n239 = case shown="无错误" w368 {
          tunnel: [200 -1] -> w369
          frame No Error {
          }
          frame Error {
          }
        }
      }
      frame "close" {
        n240 = global read "elevator 全局变量.vi" "MB session in"() -> (w381:refnum<class "MB_Master.lvclass">)
        n241 = call-dynamic "Close Session.vi"("MB session in"=w381) -> ("error out"=w380:errorcluster)  [unwired: 10 in]
      }
    }
  }
